vi "U Saturate.vi"(8 "error in (no error)":errorcluster, 10 "IMU_sample_rate":i32=200, 11 "Filtered x":dbl) -> (0 "error out":errorcluster, 3 "val out":sgl)   [LabVIEW 2014]
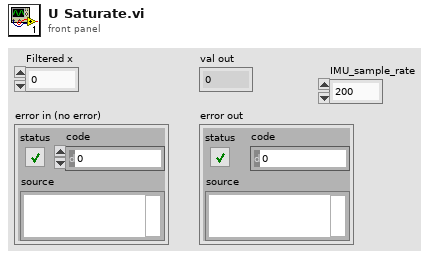
[diagram p1: front panel]
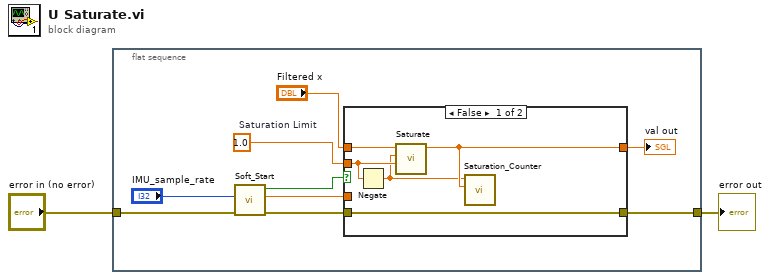
[diagram p0: block diagram]
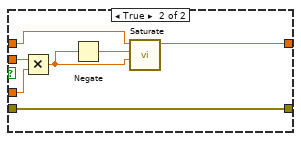
[diagram p2: hidden frame]
diagram:
  n1 = flat-sequence {
    tunnel: "error in (no error)" -> [w9]
    tunnel: [w8] -> w1
    frame #0 {
      w6 = sgl 1.0  # Saturation Limit
      n2 = call "Soft_Start.vi"("error in (no error)"=w9, "IMU_sample_rate"="IMU_sample_rate") -> ("error out"=w7:errorcluster, "Soft Start Limits"=w4:dbl, "Soft Start"=w3:bool)  [unwired: 7 in]
      n3 = case shown="False" w3 {
        tunnel: [w16 w18] -> w11
        tunnel: "Filtered x" -> [w15 w22]
        tunnel: w7 -> [w14 w23]
        tunnel: [w14 w23] -> w8
        tunnel: w6 -> [w13 w21]
        tunnel: w4 -> [_ w17]
        frame False {
          n4 = Negate(x=w13) -> (-x=w12:sgl)
          n5 = call "Saturate.vi"("Max"=w13, "Min"=w12, "X in"=w15) -> ("X out"=w16:dbl)  [unwired: 8 in]
          n6 = call "Saturation_Counter.vi"("Filtered Output"=w16, "Saturation Limit"=w12) -> ()  [unwired: 10 in]
        }
        frame True {
          n7 = Multiply(x=w21, y=w17) -> (x*y=w19:dbl)
          n8 = Negate(x=w19) -> (-x=w20:dbl)
          n9 = call "Saturate.vi"("Max"=w19, "Min"=w20, "X in"=w22) -> ("X out"=w18:dbl)  [unwired: 8 in]
        }
      }
      "val out" <- w11
    }
  }
  "error out" <- w1
